vi "Generate Random Boolean.vi"() -> (2 "Random":bool)   [LabVIEW 2015, in "Utility.lvlib"]
doc: "Generates a random boolean with equal probability for either state."
uses:
  Utility.lvlib
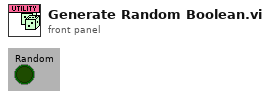
[diagram p1: front panel]
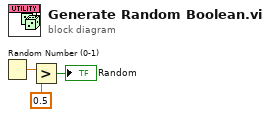
[diagram p0: block diagram]
diagram:
  n1 = Random Number (0-1)() -> (number: 0 to 1=w3:dbl)
  n2 = Greater?(x=w3, y=0.5) -> (0:→"Random":bool)
